vi "demux1-10.vi"(8 "error in":errorcluster, 10 "demux1_10(x6)_encode":T1(ring)) -> (0 "error out":errorcluster)   [LabVIEW 2018, in "MB 01 switches Module.lvlib"]
doc: "Control demux 1-10 ( AC switches)\n_____\nCreated using DQMH Event Scripter 6.0.0.122."
uses:
  MB 01 switches Module.lvlib
  demux1-10 Argument--cluster.ctl
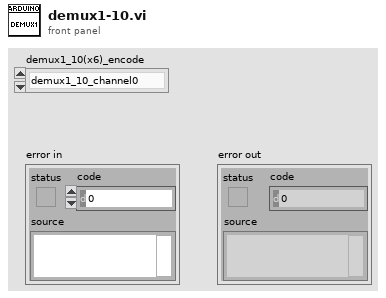
[diagram p1: front panel]
types:
  T1 = enum16{"demux1_10_channel0", "demux1_10_channel1", "demux1_10_channel2", "demux1_10_channel3", "demux1_10_channel4", "demux1_10_channel5", "demux1_10_channel6", "demux1_10_channel7", "demux1_10_channel8", "demux1_10_channel9", "demux1_10_channel10"}
  T2 = typedef "MB 01 switches Module.lvlib/demux1-10 Argument--cluster.ctl" = cluster{"demux1_10(x6)_encode":enum16{"demux1_10_channel0", "demux1_10_channel1", "demux1_10_channel2", "demux1_10_channel3", "demux1_10_channel4", "demux1_10_channel5", "demux1_10_channel6", "demux1_10_channel7", "demux1_10_channel8", "demux1_10_channel9", "demux1_10_channel10"}}
  T3 = typedef "MB 01 switches Module.lvlib/Request Events--cluster.ctl" = cluster{"Stop Module":refnum<user-event>, "Show Panel":refnum<user-event>, "Hide Panel":refnum<user-event>, "Get Module Execution Status":refnum<user-event>, "Show Diagram":refnum<user-event>, "MB01 Open":refnum<user-event>, "demux1-10":refnum<user-event>}
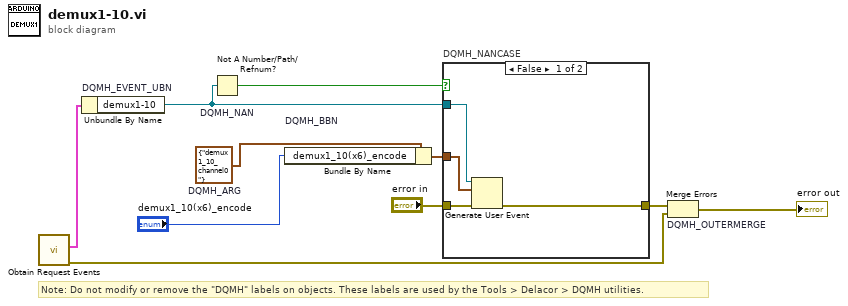
[diagram p0: block diagram]
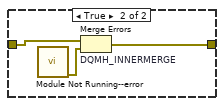
[diagram p2: hidden frame]
diagram:
  w4 = T2 {"demux1_10(x6)_encode"=enum."demux1_10_channel0"}  # DQMH_ARG
  # "Note: Do not modify or remove the \"DQMH\" labels on objects. These labels are used by the Tools > Delacor > DQMH utilities."
  n1 = call "Obtain Request Events.vi"() -> ("error out"=w2:errorcluster, "MB 01 switches Module Request Events"=w1:T3)  [unwired: 10 in]
  n2 = Unbundle By Name "DQMH_EVENT_UBN"(w1) -> ("demux1-10"=w6:refnum<user-event>)
  n3 = Not A Number/Path/Refnum? "DQMH_NAN"(number/path/refnum=w6) -> (NaN/Path/Refnum?=w7:bool)
  n4 = Bundle By Name "DQMH_BBN"(cluster=w4, "demux1_10(x6)_encode"="demux1_10(x6)_encode") -> (w8:T2)
  n5 = case "DQMH_NANCASE" shown="False" w7 {
    tunnel: "error in" -> [w14 w17]
    tunnel: [w13 w16] -> w5
    tunnel: w6 -> [w12 _]
    tunnel: w8 -> [w11 _]
    frame False {
      n6 = Generate User Event(user event=w12, event data cluster=w11, error in=w14) -> (error out=w13:errorcluster)  [unwired: 1 in, 1 out]
    }
    frame True {
      n7 = call "Module Not Running--error.vi"() -> ("error out"=w15:errorcluster)  [unwired: 11 in]
      n8 = Merge Errors "DQMH_INNERMERGE"(w17, w15) -> (w16:errorcluster)
    }
  }
  n9 = Merge Errors "DQMH_OUTERMERGE"(w5, w2) -> (→"error out":errorcluster)
